vi "WPI_DashboardNT Log FieldName Substitutions.vi"(11 "Updates in":T5(array[cluster])) -> (3 "Updates out":T5(array[cluster]))   [LabVIEW 2017]
uses:
  <vilib>/Rock Robotics/Network Tables/Protocol Operations.ctl
  <vilib>/Rock Robotics/Network Tables/Field Data.ctl
  <vilib>/Rock Robotics/Network Tables/Field Type.ctl
  <vilib>/Rock Robotics/Network Tables/Sequence.ctl
panel:
  in  "Bypass":bool
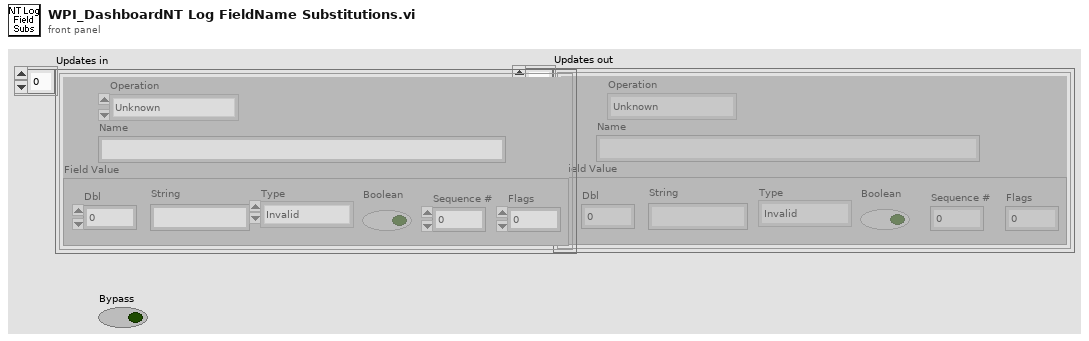
[diagram p1: front panel]
types:
  T1 = typedef "Protocol Operations.ctl" = enum16{"Unknown", "Keep Alive", "Client Hello", "Version not supported", "Server Hello Complete", "Assign", "Update", "No Op", "Server Hello", "Client Hello Complete", "Update Flags", "Delete Entry", "Delete All", "RPC Exec", "RPC Response"}
  T2 = typedef "Field Data.ctl" = cluster{"Dbl":dbl, "String":string, "Type":T3, "Boolean":bool, "Sequence #":T4, "Flags":u8}
  T3 = typedef "Field Type.ctl" = enum8{"Invalid", "Bool", "Numeric", "String", "Raw", "Boolean Array", "Numeric Array", "String Array", "RPC"}
  T4 = typedef "Sequence.ctl" = u16
  T5 = cluster{"Operation":T1, "Name":string, "Field Value":T2}[]
  T6 = cluster{"Operation":T1, "Name":string, "Field Value":T2}
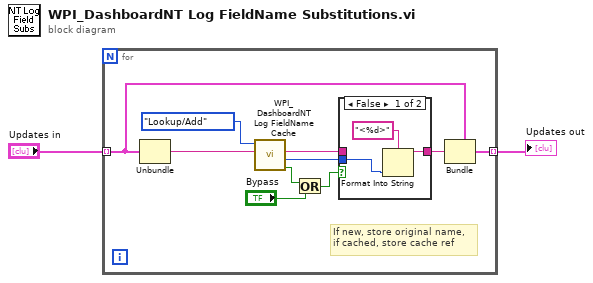
[diagram p0: block diagram]
diagram:
  n1 = for {
    tunnel: "Updates in" -> [w12] mode=indexing
    tunnel: [w6] -> w1 mode=indexing
    # "If new, store original name,\nif cached, store cache ref"
    n2 = Unbundle(w12) -> ("Name"=w11:string)  [unwired: 2 out]
    n3 = call <vilib>:"WPI_DashboardNT Log FieldName Cache.vi"("Name"=w11, "Operation"=enum16{"Lookup/Add", "Index", "Clear"}."Lookup/Add") -> ("New/Valid"=w5:bool, "Index out"=w7:i32, "Name out"=w8:string)  [unwired: 7 in]
    n4 = Or(x=w5, y="Bypass") -> (x .or. y?=w4:bool)
    n5 = case shown="False" w4 {
      tunnel: [w13 w16] -> w9
      tunnel: w8 -> [_ w16]
      tunnel: w7 -> [w14 _]
      frame False {
        n6 = Format Into String(format string="<%d>", w14) -> (resulting string=w13:string)  [unwired: 2 in, 1 out]
      }
      frame True {
      }
    }
    n7 = Bundle(cluster=w12, "Name"=w9) -> (w6:T6)  [unwired: 2 in]
  }
  "Updates out" <- w1
